vi "CMD_SERIALLIST.vi"(6 "Gantry in":refnum<class "Gantry.lvclass">, 7 "Console Log in":refnum<class "Console Log.lvclass">, 8 "error in (no error)":errorcluster, 10 "Arguments":string[](array[string]), 11 "gScript Interpreter in":refnum<class "gScript Interpreter.lvclass">) -> (0 "error out":errorcluster, 3 "gScript Interpreter out":refnum<class "gScript Interpreter.lvclass">, 4 "Gantry out":refnum<class "Gantry.lvclass">, 5 "Console Log out":refnum<class "Console Log.lvclass">)   [LabVIEW 2023, in "gScript Interpreter.lvclass"]
uses:
  gScript Interpreter.lvclass
  Shared Components/Gantry Class/Gantry.lvclass
  Application Utilities/Console Log/Console Log.lvclass
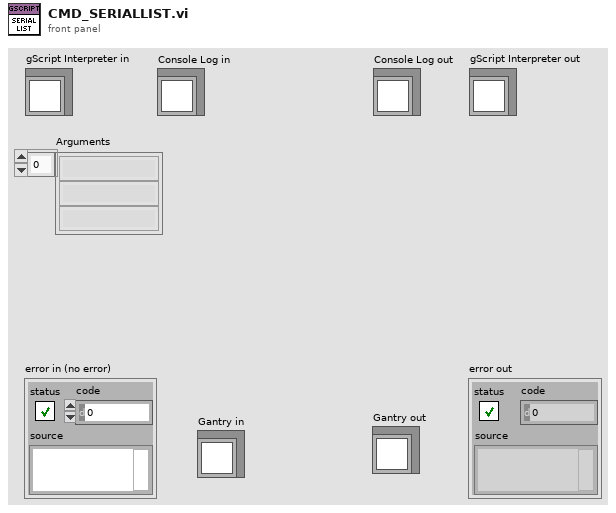
[diagram p1: front panel]
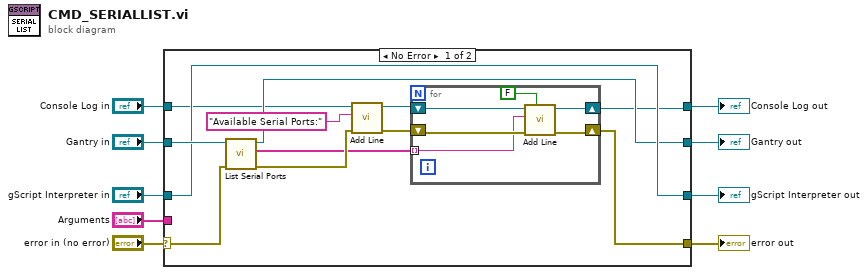
[diagram p0: block diagram]
diagram:
  n1 = case shown="No Error" "error in (no error)" {
    selector: "error in (no error)" -> [w20 w31]
    tunnel: [w11 w31] -> w8
    tunnel: [w19 w30] -> w6
    tunnel: "gScript Interpreter in" -> [w19 w30]
    tunnel: "Arguments" -> [_ _]
    tunnel: "Gantry in" -> [w21 w29]
    tunnel: [w18 w29] -> w3
    tunnel: "Console Log in" -> [w17 w28]
    tunnel: [w10 w28] -> w1
    frame No Error {
      n2 = call "List Serial Ports.vi"("error in (no error)"=w20, "Gantry in"=w21) -> ("error out"=w15:errorcluster, "find list"=w14:string[], "Gantry out"=w18:refnum<class "Gantry.lvclass">)  [unwired: 7 in]
      n3 = call "Add Line.vi"("error in"=w15, "String"="Available Serial Ports:", "Console Log in"=w17) -> ("error out"=w12:errorcluster, "Console Log out"=w13:refnum<class "Console Log.lvclass">)  [unwired: 7 in]
      n4 = for {
        tunnel: w14 -> [w24] mode=indexing
        shift-right: [w23] -> w10
        shift-left: w13 -> [w27]
        shift-right: [w22] -> w11
        shift-left: w12 -> [w25]
        n5 = call "Add Line.vi"("Timestamp"=FALSE, "error in"=w25, "String"=w24, "Console Log in"=w27) -> ("error out"=w22:errorcluster, "Console Log out"=w23:refnum<class "Console Log.lvclass">)  [unwired: 6 in]
      }
    }
    frame Error {
    }
  }
  "error out" <- w8
  "gScript Interpreter out" <- w6
  "Gantry out" <- w3
  "Console Log out" <- w1
